vi "Send Control Message.vi"(8 "error in (no error)":errorcluster, 9 "Data":variant, 10 "Msg":T1, 11 "Control Queue":refnum<queue>) -> (0 "error out":errorcluster)   [LabVIEW 2015, in "Execution.lvclass"]
uses:
  Execution.lvclass
  EXECUTION_CTRL_QUEUE_DATA.ctl
  EXECUTION_CTRL_MSG.ctl
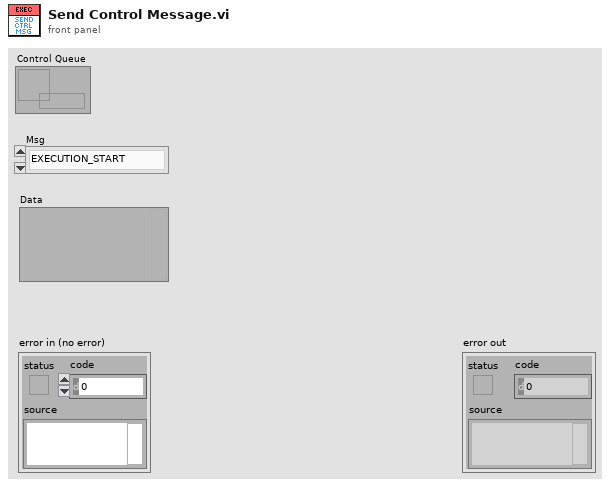
[diagram p1: front panel]
types:
  T1 = typedef "Execution.lvclass/EXECUTION_CTRL_MSG.ctl" = enum16{"EXECUTION_START", "EXECUTION_END", "EXECUTION_LOOP", "APPLICATION_STOP"}
  T2 = typedef "Execution.lvclass/EXECUTION_CTRL_QUEUE_DATA.ctl" = cluster{"Msg":T1, "Data":variant}
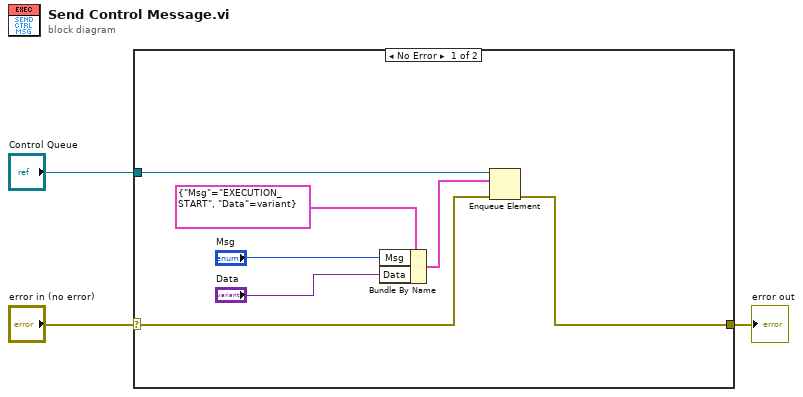
[diagram p0: block diagram]
diagram:
  n1 = case shown="No Error" "error in (no error)" {
    selector: "error in (no error)" -> [w7 w11]
    tunnel: [w6 w11] -> w2
    tunnel: "Control Queue" -> [w5 _]
    frame No Error {
      n2 = Bundle By Name(cluster=T2 {"Msg"=enum."EXECUTION_START", "Data"=variant} ("element"), "Msg"="Msg", "Data"="Data") -> (w9:T2)
      n3 = Enqueue Element(queue=w5, element=w9, error in (no error)=w7) -> (error out=w6:errorcluster)  [unwired: 1 in, 2 out]
    }
    frame Error {
    }
  }
  "error out" <- w2
